vi "Clear Tree.vi"(8 "error in (no error)":errorcluster, 11 "Tree Ref in":refnum<vi>) -> (0 "error out":errorcluster, 3 "Tree Ref out":refnum<vi>)   [LabVIEW 2017, in "Report Viewer.lvlib"]
uses:
  Report Viewer.lvlib
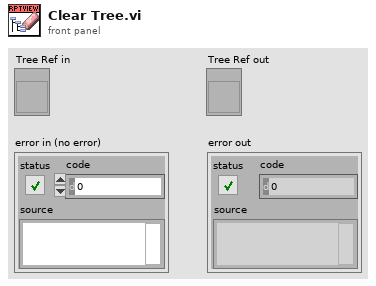
[diagram p1: front panel]
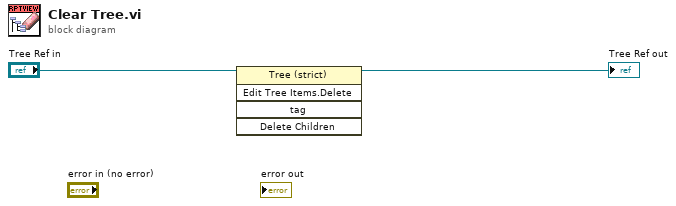
[diagram p0: block diagram]
diagram:
  n1 = invoke class="Tree (strict)" method="Edit Tree Items.Delete"(reference="Tree Ref in") -> (reference out=→"Tree Ref out":refnum<vi>)  [unwired: 4 in, 4 out]
